vi "Find Item Locations by Path.vi"(5 "Insertion point if not found":bool, 6 "Only return first found":bool, 7 "Path":string, 8 "error in (no error)":errorcluster, 10 "Offset":i32, 11 "JSON":string) -> (0 "error out":errorcluster, 1 "Items":T1[](array[typedef]))   [LabVIEW 2024, in "JSONtext.lvlib"]
uses:
  JSONtext.lvlib
  Found Items.ctl
  Parsing State.ctl
  Comma Needed for Insert.ctl
  Advance past Line Ending.vi
  Trim Whitespace__JDP.vi
  Advance past whitespace and comma.vi
  Advance past next JSON Value (inlined COPY).vi
  Advance past next JSON Scaler.vi
  Advance past String.vi
  Advance past Number.vi
  Advance past Item Name.vi
  Match Pattern.vi
  Quote and Escape JSON string.vi
  String Subset.vi
  quote and escape json string 2.vi
  Advance past Array.vi
  Advance past Object.vi
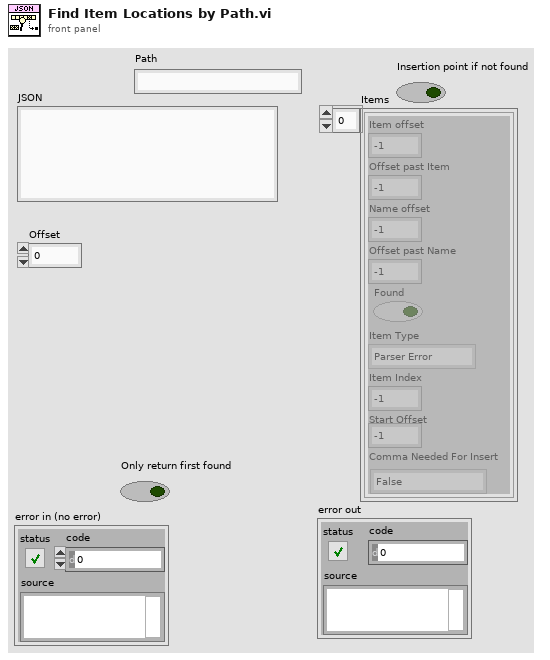
[diagram p1: front panel]
types:
  T1 = typedef "JSONtext.lvlib/Found Items.ctl" = cluster{"Item offset":i32, "Offset past Item":i32, "Name offset":i32, "Offset past Name":i32, "Found":bool, "Item Type":T2, "Item Index":i32, "Start Offset":i32, "Comma Needed For Insert":T3}
  T2 = typedef "JSONtext.lvlib/Parsing State.ctl" = enum16{"Parser Error", "Object", "Array", "String", "Number/Other", "Leading Whitespace", "Object end", "Array end", "Value end"}
  T3 = typedef "JSONtext.lvlib/Comma Needed for Insert.ctl" = enum8{"False", "True", "Following"}
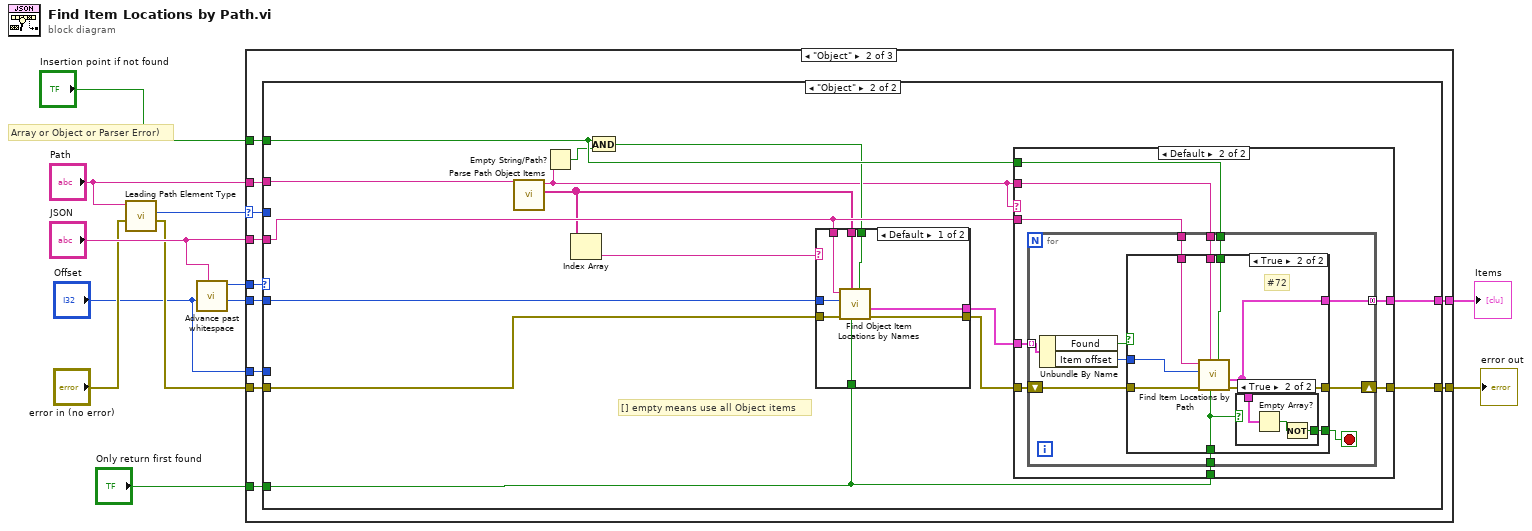
[diagram p0: block diagram]
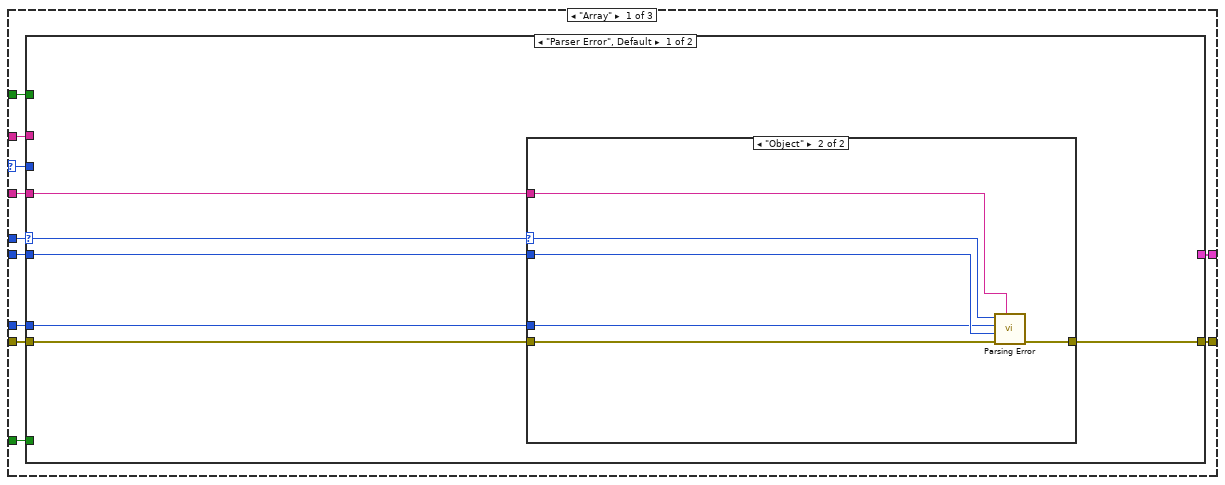
[diagram p2: hidden frame]
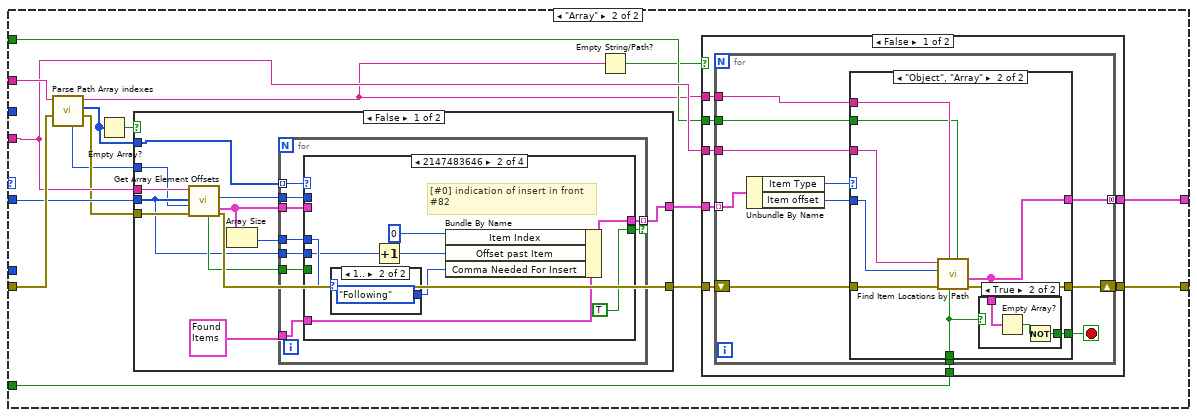
[diagram p4: hidden frame]
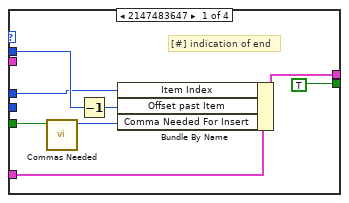
[diagram p5: hidden frame]
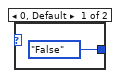
[diagram p6: hidden frame]
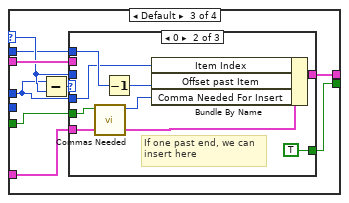
[diagram p7: hidden frame]
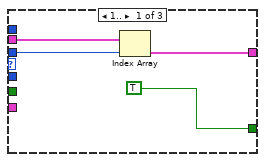
[diagram p8: hidden frame]
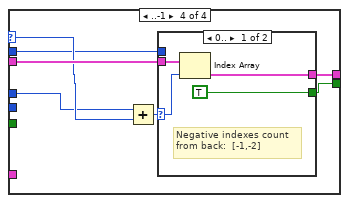
[diagram p10: hidden frame]
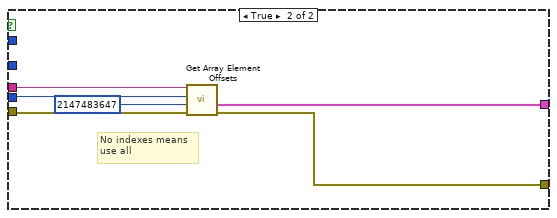
[diagram p12: hidden frame]
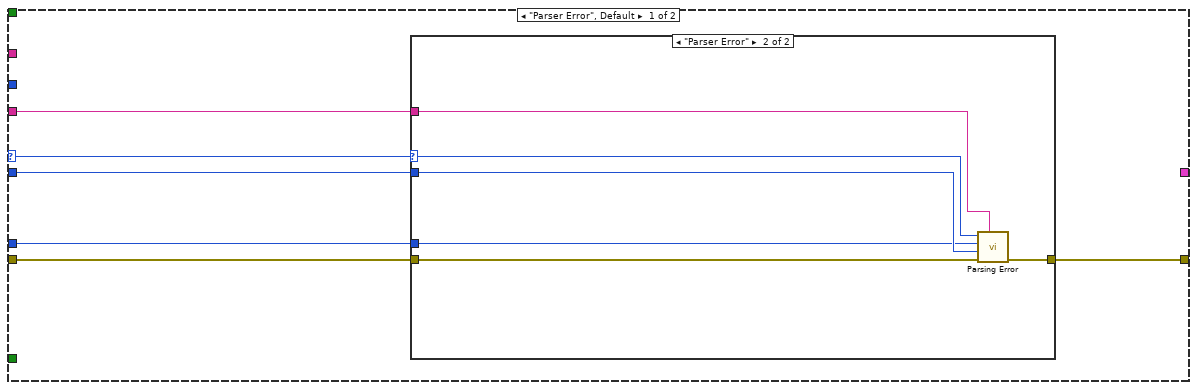
[diagram p16: hidden frame]
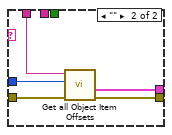
[diagram p18: hidden frame]
diagram:
  # "Array or Object or Parser Error)"
  n1 = call "Leading Path Element Type.vi"("error in (no error)"="error in (no error)", "Path"="Path") -> ("error out"=w4:errorcluster, "Path Element Type (Array or Object or Parser Error)"=w1:T2)  [unwired: 8 in]
  n2 = call "Advance past whitespace.vi"("JSON"="JSON", "Offset"="Offset") -> ("Offset of first non-whitespace"=w10:i32, "Parser State"=w3:T2)  [unwired: 7 in, 1 out]
  n3 = case shown="\"Object\"" w1 {
    selector: w1 -> [w13 w164 _]
    tunnel: [w23 w174 _] -> w12
    tunnel: "JSON" -> [w22 w173 _]
    tunnel: w10 -> [w21 w172 _]
    tunnel: [w20 w171 w250] -> w9
    tunnel: "Only return first found" -> [w19 w170 _]
    tunnel: "Insertion point if not found" -> [w18 w169 _]
    tunnel: "Path" -> [w17 w168 _]
    tunnel: w4 -> [w16 w167 w250]
    tunnel: w3 -> [w15 w166 _]
    tunnel: "Offset" -> [w14 w165 _]
    frame "Array" {
      n4 = case shown="\"Parser Error\", Default" w15 {
        selector: w15 -> [w24 _]
        tunnel: [_ w51] -> w23
        tunnel: w16 -> [w29 w48]
        tunnel: [w28 w52] -> w20
        tunnel: w17 -> [_ w49]
        tunnel: w19 -> [_ w50]
        tunnel: w18 -> [_ w45]
        tunnel: w21 -> [w27 w47]
        tunnel: w22 -> [w26 w46]
        tunnel: w14 -> [w25 _]
        tunnel: w13 -> [_ _]
        frame "Parser Error", Default {
          n5 = case shown="\"Object\"" w24 {
            selector: w24 -> [_ w31]
            tunnel: w29 -> [w30 w36]
            tunnel: [w30 w35] -> w28
            tunnel: w27 -> [_ w34]
            tunnel: w26 -> [_ w33]
            tunnel: w25 -> [_ w32]
            frame "Parser Error", Default {
            }
            frame "Object" {
              n6 = call "Parsing Error.vi"("JSON"=w33, "error in (no error)"=w36, "Offset past match"=w34, "Value start"=w32, "State"=w31) -> ("error out"=w35:errorcluster)  [unwired: 6 in]
            }
          }
        }
        frame "Array" {
          n7 = call "Parse Path Array indexes.vi"("error in (no error)"=w48, "Path with leading Array element"=w49) -> ("error out"=w39:errorcluster, "Indexes (empty means use all)"=w40:i32[], "Rest or Path"=w44:string, "Max Index to parse"=w37:i32)  [unwired: 6 in]
          n8 = Empty Array?(array=w40) -> (empty?=w42:bool)
          n9 = case shown="False" w42 {
            tunnel: [w64 w125] -> w41
            tunnel: w40 -> [w57 _]
            tunnel: w39 -> [w62 w127]
            tunnel: w47 -> [w53 w128]
            tunnel: w46 -> [w61 w129]
            tunnel: [w60 w126] -> w38
            tunnel: w37 -> [w54 _]
            frame False {
              n10 = call "Get Array Element Offsets.vi"("error in (no error)"=w62, "Max Index"=w54, "Offset"=w53, "JSON"=w61) -> ("error out"=w60:errorcluster, "Elements"=w59:T1[], "Offset past Array"=w58:i32, "Comma Needed for Insert"=w56:bool)  [unwired: 4 in]
              n11 = Array Size(array=w59) -> (size(s)=w63:i32)
              n12 = for {
                tunnel: w57 -> [w71] mode=indexing
                tunnel: w59 -> [w73]
                tunnel: [w72] -> w64 mode=indexing if=w68
                tunnel: w63 -> [w70]
                tunnel: w58 -> [w69]
                tunnel: w56 -> [w67]
                tunnel: T1 {"Item offset"=0, "Offset past Item"=0, "Name offset"=0, "Offset past Name"=0, "Found"=FALSE, "Item Type"=enum."Parser Error", "Item Index"=0, "Start Offset"=0, "Comma Needed For Insert"=enum."False"} -> [w66]
                tunnel: w53 -> [w65]
                n13 = case shown="2147483646" w71 {
                  selector: w71 -> [_ _ w98 w117]
                  tunnel: w73 -> [_ _ w100 w119]
                  tunnel: [w81 w89 w99 w118] -> w72
                  tunnel: w70 -> [w77 w83 w94 w113]
                  tunnel: [TRUE TRUE w97 w116] -> w68
                  tunnel: w69 -> [w80 _ w95 w114]
                  tunnel: w66 -> [w76 w86 w93 _]
                  tunnel: w67 -> [w75 _ w92 _]
                  tunnel: w65 -> [_ w82 _ _]
                  frame 2147483647 {
                    # "[#] indication of end"
                    n14 = call "Commas Needed.vi"("Comma needed"=w75) -> ("Comma Needed For Insert"=w74:T3)  [unwired: 10 in]
                    n15 = Decrement(x=w80) -> (x-1=w79:i32)
                    n16 = Bundle By Name(cluster=w76, "Item Index"=w77, "Offset past Item"=w79, "Comma Needed For Insert"=w74) -> (w81:T1)
                  }
                  frame 2147483646 {
                    # "[#0] indication of insert in front\n#82"
                    n17 = case shown="1.." w83 {
                      tunnel: [Comma_Needed_for_Insert."False" ("Comma Needed For Insert") Comma_Needed_for_Insert."Following" ("Comma Needed For Insert")] -> w84
                      frame 0, Default {
                      }
                      frame 1.. {
                      }
                    }
                    n18 = Increment(x=w82) -> (x+1=w88:i32)
                    n19 = Bundle By Name(cluster=w86, "Item Index"=0, "Offset past Item"=w88, "Comma Needed For Insert"=w84) -> (w89:T1)
                  }
                  frame Default {
                    n20 = Subtract(x=w94, y=w98) -> (x-y=w96:i32)
                    n21 = case shown="0" w96 {
                      tunnel: w100 -> [w104 _ _]
                      tunnel: [w103 w110 _] -> w99
                      tunnel: w98 -> [w102 _ _]
                      tunnel: [TRUE TRUE _] -> w97
                      tunnel: w95 -> [_ w109 _]
                      tunnel: w94 -> [_ w107 _]
                      tunnel: w93 -> [_ w108 _]
                      tunnel: w92 -> [_ w106 _]
                      frame 1.. {
                        n22 = Index Array(array=w104, index=w102) -> (element=w103:T1)
                      }
                      frame 0 {
                        # "If one past end, we can\ninsert here"
                        n23 = call "Commas Needed.vi"("Comma needed"=w106) -> ("Comma Needed For Insert"=w105:T3)  [unwired: 10 in]
                        n24 = Decrement(x=w109) -> (x-1=w112:i32)
                        n25 = Bundle By Name(cluster=w108, "Item Index"=w107, "Offset past Item"=w112, "Comma Needed For Insert"=w105) -> (w110:T1)
                      }
                      frame Default {
                      }
                    }
                  }
                  frame ..-1 {
                    n26 = Add(x=w113, y=w117) -> (x+y=w115:i32)
                    n27 = case shown="0.." w115 {
                      selector: w115 -> [w120 _]
                      tunnel: w119 -> [w123 _]
                      tunnel: [w122 _] -> w118
                      tunnel: [TRUE _] -> w116
                      tunnel: w114 -> [_ _]
                      frame 0.. {
                        # "Negative indexes count\nfrom back:  [-1,-2]"
                        n28 = Index Array(array=w123, index=w120) -> (element=w122:T1)
                      }
                      frame Default {
                      }
                    }
                  }
                }
              }
            }
            frame True {
              # "No indexes means\nuse all"
              n29 = call "Get Array Element Offsets.vi"("error in (no error)"=w127, "Max Index"=2147483647, "Offset"=w128, "JSON"=w129) -> ("error out"=w126:errorcluster, "Elements"=w125:T1[])  [unwired: 4 in, 2 out]
            }
          }
          n30 = Empty String/Path?(string/path=w44) -> (empty?=w43:bool)
          n31 = case shown="False" w43 {
            tunnel: [w137 w163] -> w52
            tunnel: [w136 w162] -> w51
            tunnel: w41 -> [w135 w162]
            tunnel: w38 -> [w134 w163]
            tunnel: w46 -> [w133 _]
            tunnel: w50 -> [w132 _]
            tunnel: w44 -> [w131 _]
            tunnel: w45 -> [w130 _]
            frame False {
              n32 = for {
                tunnel: [w146] -> w136 mode=concatenating
                shift-right: [w147] -> w137
                shift-left: w134 -> [w148]
                tunnel: w131 -> [w145]
                tunnel: w135 -> [w144] mode=indexing
                tunnel: w133 -> [w142]
                tunnel: w132 -> [w140]
                tunnel: w130 -> [w138]
                stop <- w139 stop-if-true
                n33 = Unbundle By Name(w144) -> ("Item Type"=w143:T2, "Item offset"=w141:i32)
                n34 = case shown="\"Object\", \"Array\"" w143 {
                  tunnel: w148 -> [w149 w158]
                  tunnel: [w149 w157] -> w147
                  tunnel: [_ w153] -> w146
                  tunnel: w145 -> [_ w156]
                  tunnel: w142 -> [_ w155]
                  tunnel: w141 -> [_ w154]
                  tunnel: w140 -> [_ w151]
                  tunnel: [_ w152] -> w139
                  tunnel: w138 -> [_ w150]
                  frame "Parser Error", Default {
                  }
                  frame "Object", "Array" {
                    n35 = call "Find Item Locations by Path.vi"("Insertion point if not found"=w150, "Only return first found"=w151, "Path"=w156, "error in (no error)"=w158, "Offset"=w154, "JSON"=w155) -> ("error out"=w157:errorcluster, "Items"=w153:T1[])  [unwired: 4 in]
                    n36 = case shown="True" w151 {
                      tunnel: w153 -> [_ w161]
                      tunnel: [_ w159] -> w152
                      frame False {
                      }
                      frame True {
                        n37 = Empty Array?(array=w161) -> (empty?=w160:bool)
                        n38 = Not(x=w160) -> (.not. x?=w159:bool)
                      }
                    }
                  }
                }
              }
            }
            frame True {
            }
          }
        }
      }
    }
    frame "Object" {
      n39 = case shown="\"Object\"" w166 {
        selector: w166 -> [w175 _]
        tunnel: [_ w201] -> w174
        tunnel: w167 -> [w180 w199]
        tunnel: [w179 w202] -> w171
        tunnel: w168 -> [_ w198]
        tunnel: w170 -> [_ w196]
        tunnel: w169 -> [_ w195]
        tunnel: w172 -> [w178 w197]
        tunnel: w173 -> [w177 w200]
        tunnel: w165 -> [w176 _]
        tunnel: w164 -> [_ _]
        frame "Parser Error", Default {
          n40 = case shown="\"Parser Error\"" w175 {
            selector: w175 -> [_ w182]
            tunnel: w180 -> [w181 w187]
            tunnel: [w181 w186] -> w179
            tunnel: w178 -> [_ w185]
            tunnel: w177 -> [_ w184]
            tunnel: w176 -> [_ w183]
            frame Default {
            }
            frame "Parser Error" {
              n41 = call "Parsing Error.vi"("JSON"=w184, "error in (no error)"=w187, "Offset past match"=w185, "Value start"=w183, "State"=w182) -> ("error out"=w186:errorcluster)  [unwired: 6 in]
            }
          }
        }
        frame "Object" {
          # "[] empty means use all Object items"
          n42 = call "Parse Path Object Items.vi"("Path with leading Object element"=w198) -> ("<JSON>items names"=w192:string[], "Rest or Path"=w188:string)  [unwired: 7 in, 2 out]
          n43 = Empty String/Path?(string/path=w188) -> (empty?=w189:bool)
          n44 = Index Array(array=w192) -> (element=w191:string)  [unwired: 1 in]
          n45 = And(x=w195, y=w189) -> (x .and. y?=w190:bool)
          n46 = case shown="Default" w191 {
            tunnel: w200 -> [w210 w215]
            tunnel: w199 -> [w209 w213]
            tunnel: w197 -> [w208 w214]
            tunnel: w192 -> [w207 _]
            tunnel: [w206 w212] -> w194
            tunnel: [w205 w211] -> w193
            tunnel: w196 -> [w204 _]
            tunnel: w190 -> [w203 _]
            frame Default {
              n47 = call "Find Object Item Locations by Names.vi"("Insertion point if not found"=w203, "Only return first found"=w204, "Item Names <JSON>"=w207, "error in (no error)"=w209, "Object Offset"=w208, "JSON"=w210) -> ("error out"=w206:errorcluster, "Items"=w205:T1[])  [unwired: 4 in]
            }
            frame "" {
              n48 = call "Get all Object Item Offsets.vi"("error in (no error)"=w213, "Offset"=w214, "JSON"=w215) -> ("error out"=w212:errorcluster, "Items"=w211:T1[])  [unwired: 6 in, 1 out]
            }
          }
          n49 = case shown="Default" w188 {
            tunnel: [w216 w225] -> w202
            tunnel: [w217 w224] -> w201
            tunnel: w200 -> [_ w223]
            tunnel: w188 -> [_ w222]
            tunnel: w194 -> [w216 w221]
            tunnel: w193 -> [w217 w220]
            tunnel: w196 -> [_ w219]
            tunnel: w195 -> [_ w218]
            frame "" {
            }
            frame Default {
              n50 = for {
                tunnel: [w235] -> w224 mode=concatenating
                tunnel: w223 -> [w234]
                tunnel: w222 -> [w233]
                tunnel: w220 -> [w231] mode=indexing
                shift-right: [w236] -> w225
                shift-left: w221 -> [w232]
                tunnel: w219 -> [w228]
                tunnel: w218 -> [w226]
                stop <- w227 stop-if-true
                n51 = Unbundle By Name(w231) -> ("Found"=w230:bool, "Item offset"=w229:i32)
                n52 = case shown="True" w230 {
                  tunnel: [w237 w246] -> w236
                  tunnel: [_ w240] -> w235
                  tunnel: w234 -> [_ w245]
                  tunnel: w233 -> [_ w244]
                  tunnel: w232 -> [w237 w243]
                  tunnel: w229 -> [_ w242]
                  tunnel: w228 -> [_ w241]
                  tunnel: [_ w239] -> w227
                  tunnel: w226 -> [_ w238]
                  frame False {
                  }
                  frame True {
                    # "#72"
                    n53 = call "Find Item Locations by Path.vi"("Insertion point if not found"=w238, "Only return first found"=w241, "Path"=w244, "error in (no error)"=w243, "Offset"=w242, "JSON"=w245) -> ("error out"=w246:errorcluster, "Items"=w240:T1[])  [unwired: 4 in]
                    n54 = case shown="True" w241 {
                      tunnel: w240 -> [_ w249]
                      tunnel: [_ w247] -> w239
                      frame False {
                      }
                      frame True {
                        n55 = Empty Array?(array=w249) -> (empty?=w248:bool)
                        n56 = Not(x=w248) -> (.not. x?=w247:bool)
                      }
                    }
                  }
                }
              }
            }
          }
        }
      }
    }
    frame "Parser Error", Default {
    }
  }
  "Items" <- w12
  "error out" <- w9
